vi "AODO-Clear Tasks.vi"(0 "Config":T3, 5 "AO Tasks":T2[](array[typedef]), 9 "DO Tasks":T1) -> (15 "error out":errorcluster)   [LabVIEW 2020]
uses:
  Typedefs/AODO-Config.ctl
  Typedefs/AODO-Output Spec.ctl
  Typedefs/DO-Output Spec.ctl
  Typedefs/AODO-Task Specification.ctl
  Typedefs/AODO-DO Tasks.ctl
  <resource>/objmgr/daqmx.rc
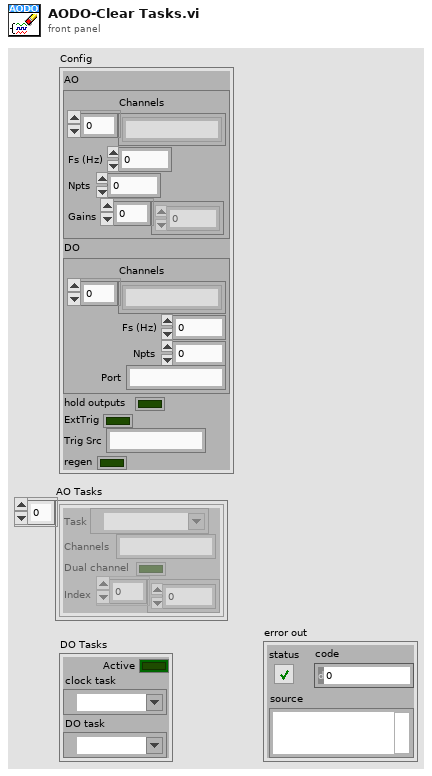
[diagram p1: front panel]
types:
  T1 = typedef "AODO-DO Tasks.ctl" = cluster{"Active":bool, "clock task":refnum<k21>, "DO task":refnum<k21>}
  T2 = typedef "AODO-Task Specification.ctl" = cluster{"Task":refnum<k21>, "Channels":string, "Dual channel":bool, "Index":i32[]}
  T3 = typedef "AODO-Config.ctl" = cluster{"AO":T4, "DO":T5, "hold outputs":bool, "ExtTrig":bool, "Trig Src":string, "regen":bool}
  T4 = typedef "AODO-Output Spec.ctl" = cluster{"Channels":string[], "Fs (Hz)":dbl, "Npts":i32, "Gains":dbl[]}
  T5 = typedef "DO-Output Spec.ctl" = cluster{"Channels":string[], "Fs (Hz)":dbl, "Npts":i32, "Port":string}
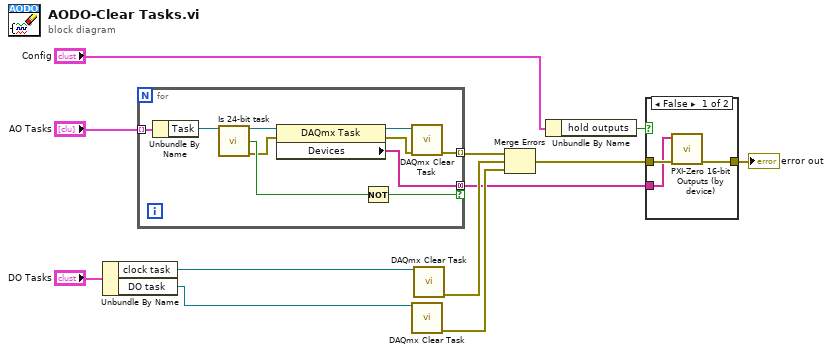
[diagram p0: block diagram]
diagram:
  n1 = Unbundle By Name("DO Tasks") -> ("clock task"=w9:refnum<k21>, "DO task"=w10:refnum<k21>)
  n2 = for {
    tunnel: "AO Tasks" -> [w22] mode=indexing
    tunnel: [w21] -> w5 mode=indexing
    tunnel: [w17] -> w1 mode=concatenating if=w16
    n3 = Unbundle By Name(w22) -> ("Task"=w19:refnum<k21>)
    n4 = call "Is 24-bit task.vi"("task"=w19) -> ("task out"=w18:refnum<k21>, "is 24bit?"=w15:bool, "error out"=w14:errorcluster)  [unwired: 9 in, 3 out]
    n5 = property class="DAQmx Task"(reference=w18, error in=w14) -> (reference out=w20:refnum<k21>, error out=w13:errorcluster, "Devices"=w17:tag[])
    n6 = Not(x=w15) -> (.not. x?=w16:bool)
    n7 = call <vilib>:"DAQmx Clear Task.vi"("task in"=w20, "error in"=w13) -> ("error out"=w21:errorcluster)  [unwired: 13 in]
  }
  n8 = call <vilib>:"DAQmx Clear Task.vi"("task in"=w10) -> ("error out"=w3:errorcluster)  [unwired: 14 in]
  n9 = call <vilib>:"DAQmx Clear Task.vi"("task in"=w9) -> ("error out"=w4:errorcluster)  [unwired: 14 in]
  n10 = Merge Errors(w5, w4, w3) -> (w2:errorcluster)
  n11 = Unbundle By Name("Config") -> ("hold outputs"=w6:bool)
  n12 = case shown="False" w6 {
    tunnel: w2 -> [w25 w26]
    tunnel: [w24 w26] -> w7
    tunnel: w1 -> [w23 _]
    frame False {
      n13 = call "PXI-Zero 16-bit Outputs (by device).vi"("error in (no error)"=w25, "DevNames"=w23) -> ("error out"=w24:errorcluster)  [unwired: 9 in]
    }
    frame True {
    }
  }
  "error out" <- w7
